vi "escribe_tbl_ajuste_previo.vi"(8 "error in (no error)":errorcluster, 11 "DB in":refnum<class "Base de Datos.lvclass">) -> (0 "error out":errorcluster, 2 "last_id_ajuste_previo":string, 3 "object out":refnum<class "Base de Datos.lvclass">)   [LabVIEW 2019, in "Base de Datos.lvclass"]
uses:
  Base de Datos.lvclass
  Base de Datos.lvclass/Base de Datos.ctl
  SQLiteConnector/SQLiteConnection.lvclass
panel:
  out "Paso 1":string
  # "Tabla que registra los datos de los ajustes previos"
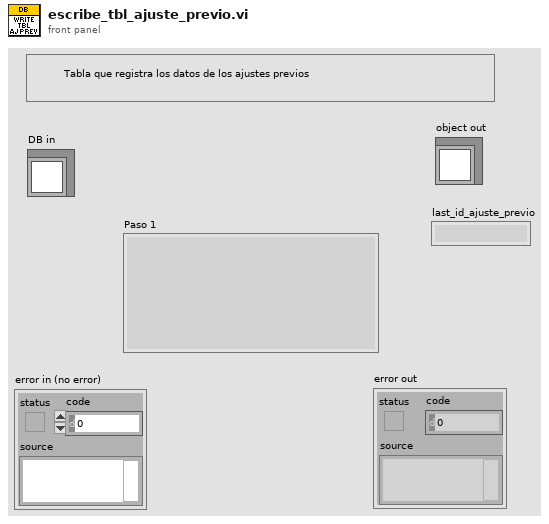
[diagram p1: front panel]
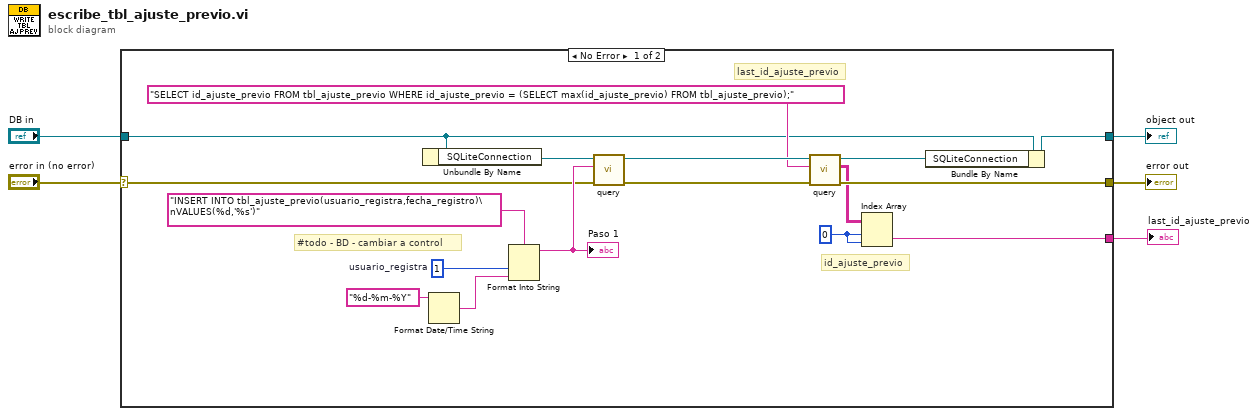
[diagram p0: block diagram]
diagram:
  n1 = case shown="No Error" "error in (no error)" {
    selector: "error in (no error)" -> [w16 w24]
    tunnel: [w15 w24] -> w5
    tunnel: "DB in" -> [w9 w23]
    tunnel: [w10 _] -> w2
    tunnel: [w7 w23] -> w1
    frame No Error {
      w12 = 0 ("index (row)")
      w18 = 1  # usuario_registra
      # "id_ajuste_previo"
      # "last_id_ajuste_previo"
      # "#todo - BD - cambiar a control"
      n2 = Unbundle By Name(w9) -> ("SQLiteConnection"=w8:refnum<class "SQLiteConnection.lvclass">)
      n3 = Format Date/Time String(time format string (%c)="%d-%m-%Y") -> (date/time string=w17:string)  [unwired: 2 in]
      n4 = Format Into String(format string="INSERT INTO tbl_ajuste_previo(usuario_registra,fecha_registro)\nVALUES(%d,'%s')", w18, w17) -> (resulting string=w22:string)  [unwired: 2 in, 1 out]
      "Paso 1" <- w22
      n5 = call "query.vi"("error in (no error)"=w16, "SQL Statement"=w22, "object in"=w8) -> ("error out"=w19:errorcluster, "object out"=w14:refnum<class "SQLiteConnection.lvclass">)  [unwired: 5 in, 2 out]
      n6 = call "query.vi"("error in (no error)"=w19, "SQL Statement"="SELECT id_ajuste_previo FROM tbl_ajuste_previo WHERE id_ajuste_previo = (SELECT max(id_ajuste_previo) FROM tbl_ajuste_previo);" ("format string"), "object in"=w14) -> ("error out"=w15:errorcluster, "result"=w11:string[][], "object out"=w6:refnum<class "SQLiteConnection.lvclass">)  [unwired: 5 in, 1 out]
      n7 = Index Array(array=w11, index (row)=w12, index (col)=w12) -> (element=w10:string)
      n8 = Bundle By Name(cluster=w9, "SQLiteConnection"=w6) -> (w7:refnum<class "Base de Datos.lvclass">)
    }
    frame Error {
    }
  }
  "error out" <- w5
  "object out" <- w1
  "last_id_ajuste_previo" <- w2
